vi "Open CITI File.vi"(8 "error in (no error)":errorcluster, 11 "CITI File Path":path) -> (0 "error out":errorcluster, 3 "CITI reference out":refnum<k24>)   [LabVIEW 2023, in "NI_HFNetworkAnalysis.lvlib"]
doc: "Open a reference to the specified CITI file and load all CITI packages into memory.\n\n<b>Note</b>\nUse <b>Get CITI Packages.vi</b> to retrieve the CITI packages from the referenced file."
uses:
  NI_HFNetworkAnalysis.lvlib
  C:/srd-semi-rfcal-software/AuxTools/STSRFFixtureCharactUtility/Source/Code Modules/Fixture/Dependencies/HFNetworkAnalysis/Support Files/NACE.Utils.Data.dll
  Support Files/NACE.Utils.Data.dll
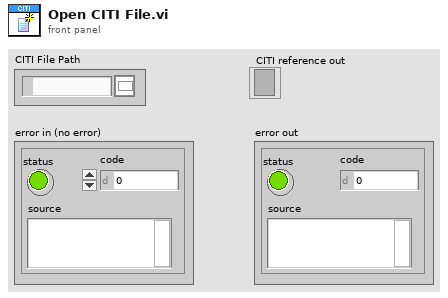
[diagram p1: front panel]
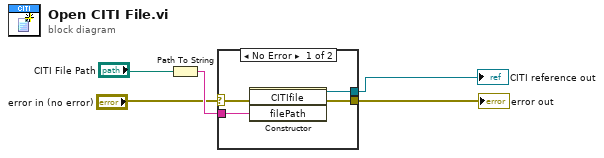
[diagram p0: block diagram]
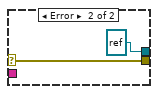
[diagram p2: hidden frame]
diagram:
  n1 = Path To String(path="CITI File Path") -> (string=w5:string)
  n2 = case shown="No Error" "error in (no error)" {
    selector: "error in (no error)" -> [w9 w11]
    tunnel: w5 -> [w8 _]
    tunnel: [w7 w11] -> w1
    tunnel: [w6 refnum<k24> refnum ("new reference")] -> w4
    frame No Error {
      n3 = constructor class="CITIfile"(error in=w9, "filePath"=w8) -> (reference out=w6:refnum<k24>, error out=w7:errorcluster)  [unwired: 2 in, 2 out]
    }
    frame Error {
    }
  }
  "error out" <- w1
  "CITI reference out" <- w4
